vi "Write userEventPeriod.vi"(8 "error in (no error)":errorcluster, 10 "userEventPeriod":refnum<user-event>, 11 "WindowsTarget in":refnum<class "WindowsTarget.lvclass">) -> (0 "error out":errorcluster, 3 "WindowsTarget out":refnum<class "WindowsTarget.lvclass">)   [LabVIEW 2012, in "WindowsTarget.lvclass"]
uses:
  WindowsTarget.lvclass
  WindowsTarget.lvclass/WindowsTarget.ctl
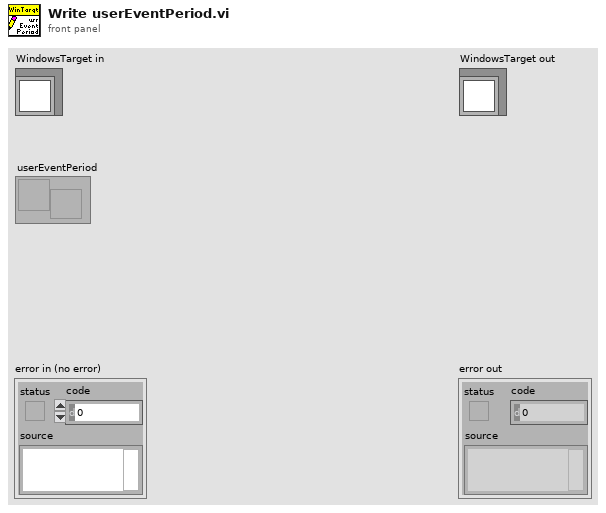
[diagram p1: front panel]
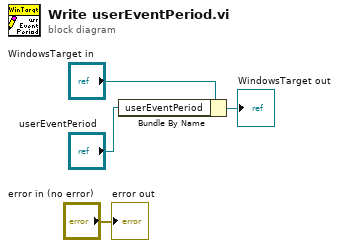
[diagram p0: block diagram]
diagram:
  n1 = Bundle By Name(cluster="WindowsTarget in", "userEventPeriod"="userEventPeriod") -> (→"WindowsTarget out":refnum<class "WindowsTarget.lvclass">)
  "error out" <- "error in (no error)"
